vi "HFRR ADV v030 new software.vi"() -> ()   [LabVIEW 2025] (continued)
        n1482 = property on="About" class="Bool (strict)"("DisabledEnum"=w1363) -> ()  [unwired: 2 in, 2 out]
      }
      frame "Test Setup" {
        w1369 = T19."Enabled" ("Disabled")
        n1483 = local read "Service Password enable"() -> (w1368:bool)
        n1484 = property on="Dashboard" class="Bool (strict)"("DisabledEnum"=T19."Disabled" ("Disabled")) -> ()  [unwired: 2 in, 2 out]
        n1485 = property on="Imaging" class="Bool (strict)"("DisabledEnum"=w1369) -> ()  [unwired: 2 in, 2 out]
        n1486 = property on="Analysis" class="Bool (strict)"("DisabledEnum"=w1369) -> ()  [unwired: 2 in, 2 out]
        n1487 = property on="Home" class="Bool (strict)"("DisabledEnum"=w1369) -> ()  [unwired: 2 in, 2 out]
        n1488 = property on="Report" class="Bool (strict)"("DisabledEnum"=w1369) -> ()  [unwired: 2 in, 2 out]
        n1489 = property on="Test Setup" class="Bool (strict)"("DisabledEnum"=w1369) -> ()  [unwired: 2 in, 2 out]
        n1490 = case shown="True" w1368 {
          tunnel: [T19."Disabled" ("Disabled") T19."Enabled" ("Disabled")] -> w1367
          frame False {
          }
          frame True {
          }
        }
        n1491 = property on="About" class="Bool (strict)"("DisabledEnum"=w1367) -> ()  [unwired: 2 in, 2 out]
      }
      frame "Adv Scar" {
        w1376 = T19."Enabled" ("Disabled")
        n1492 = property on="Dashboard" class="Bool (strict)"("DisabledEnum"=T19."Disabled" ("Disabled")) -> ()  [unwired: 2 in, 2 out]
        n1493 = property on="Imaging" class="Bool (strict)"("DisabledEnum"=w1376) -> ()  [unwired: 2 in, 2 out]
        n1494 = property on="Analysis" class="Bool (strict)"("DisabledEnum"=w1376) -> ()  [unwired: 2 in, 2 out]
        n1495 = property on="Home" class="Bool (strict)"("DisabledEnum"=w1376) -> ()  [unwired: 2 in, 2 out]
        n1496 = property on="Report" class="Bool (strict)"("DisabledEnum"=w1376) -> ()  [unwired: 2 in, 2 out]
        n1497 = property on="Test Setup" class="Bool (strict)"("DisabledEnum"=w1376) -> ()  [unwired: 2 in, 2 out]
        n1498 = local read "Service Password enable"() -> (w1374:bool)
        n1499 = case shown="True" w1374 {
          tunnel: [T19."Disabled" ("Disabled") T19."Enabled" ("Disabled")] -> w1373
          frame False {
          }
          frame True {
          }
        }
        n1500 = property on="About" class="Bool (strict)"("DisabledEnum"=w1373) -> ()  [unwired: 2 in, 2 out]
      }
      frame "Calibration" {
        w1379 = T19."Enabled" ("Disabled")
        n1501 = property on="Dashboard" class="Bool (strict)"("DisabledEnum"=T19."Disabled" ("Disabled")) -> ()  [unwired: 2 in, 2 out]
        n1502 = property on="Imaging" class="Bool (strict)"("DisabledEnum"=w1379) -> ()  [unwired: 2 in, 2 out]
        n1503 = property on="Analysis" class="Bool (strict)"("DisabledEnum"=w1379) -> ()  [unwired: 2 in, 2 out]
        n1504 = property on="Home" class="Bool (strict)"("DisabledEnum"=w1379) -> ()  [unwired: 2 in, 2 out]
        n1505 = property on="Report" class="Bool (strict)"("DisabledEnum"=w1379) -> ()  [unwired: 2 in, 2 out]
        n1506 = property on="Test Setup" class="Bool (strict)"("DisabledEnum"=w1379) -> ()  [unwired: 2 in, 2 out]
        n1507 = local read "Service Password enable"() -> (w1381:bool)
        n1508 = property on="Calibration" class="Bool (strict)"("DisabledEnum"=w1379) -> ()  [unwired: 2 in, 2 out]
        n1509 = case shown="True" w1381 {
          tunnel: [T19."Disabled" ("Disabled") T19."Enabled" ("Disabled")] -> w1380
          frame False {
          }
          frame True {
          }
        }
        n1510 = property on="About" class="Bool (strict)"("DisabledEnum"=w1380) -> ()  [unwired: 2 in, 2 out]
      }
      frame "Adv Scar Report" {
        w1387 = T19."Enabled" ("Disabled")
        n1511 = property on="Dashboard" class="Bool (strict)"("DisabledEnum"=T19."Disabled" ("Disabled")) -> ()  [unwired: 2 in, 2 out]
        n1512 = property on="Imaging" class="Bool (strict)"("DisabledEnum"=w1387) -> ()  [unwired: 2 in, 2 out]
        n1513 = property on="Analysis" class="Bool (strict)"("DisabledEnum"=w1387) -> ()  [unwired: 2 in, 2 out]
        n1514 = property on="Home" class="Bool (strict)"("DisabledEnum"=w1387) -> ()  [unwired: 2 in, 2 out]
        n1515 = property on="Report" class="Bool (strict)"("DisabledEnum"=w1387) -> ()  [unwired: 2 in, 2 out]
        n1516 = property on="Test Setup" class="Bool (strict)"("DisabledEnum"=w1387) -> ()  [unwired: 2 in, 2 out]
        n1517 = local read "Service Password enable"() -> (w1386:bool)
        n1518 = case shown="True" w1386 {
          tunnel: [T19."Disabled" ("Disabled") T19."Enabled" ("Disabled")] -> w1385
          frame False {
          }
          frame True {
          }
        }
        n1519 = property on="About" class="Bool (strict)"("DisabledEnum"=w1385) -> ()  [unwired: 2 in, 2 out]
      }
      frame "Compare Files" {
        w1393 = T19."Enabled" ("Disabled")
        n1520 = local read "Service Password enable"() -> (w1392:bool)
        n1521 = property on="Dashboard" class="Bool (strict)"("DisabledEnum"=T19."Disabled" ("Disabled")) -> ()  [unwired: 2 in, 2 out]
        n1522 = property on="Imaging" class="Bool (strict)"("DisabledEnum"=w1393) -> ()  [unwired: 2 in, 2 out]
        n1523 = property on="Analysis" class="Bool (strict)"("DisabledEnum"=w1393) -> ()  [unwired: 2 in, 2 out]
        n1524 = property on="Home" class="Bool (strict)"("DisabledEnum"=w1393) -> ()  [unwired: 2 in, 2 out]
        n1525 = property on="Report" class="Bool (strict)"("DisabledEnum"=w1393) -> ()  [unwired: 2 in, 2 out]
        n1526 = property on="Test Setup" class="Bool (strict)"("DisabledEnum"=w1393) -> ()  [unwired: 2 in, 2 out]
        n1527 = case shown="True" w1392 {
          tunnel: [T19."Disabled" ("Disabled") T19."Enabled" ("Disabled")] -> w1391
          frame False {
          }
          frame True {
          }
        }
        n1528 = property on="About" class="Bool (strict)"("DisabledEnum"=w1391) -> ()  [unwired: 2 in, 2 out]
      }
      frame "Acquire" {
        n1529 = local read "Service Password enable"() -> (w1398:bool)
        n1530 = property on="Test Setup" class="Bool (strict)"("DisabledEnum"=T19."Disabled" ("Disabled")) -> ()  [unwired: 2 in, 2 out]
        n1531 = local read "Auto Start Test"() -> (w1400:bool)
        n1532 = local read "RUN"() -> (w1402:bool)
        n1533 = case shown="True" w1398 {
          tunnel: [T19."Disabled" ("Disabled") T19."Enabled" ("Disabled")] -> w1399
          frame False {
          }
          frame True {
          }
        }
        n1534 = Or(x=w1402, y=w1400) -> (x .or. y?=w1401:bool)
        n1535 = case shown="True" w1401 {
          tunnel: [T19."Enabled" ("Disabled") T19."Disabled" ("Disabled")] -> w1397
          frame False {
          }
          frame True {
          }
        }
        n1536 = property on="About" class="Bool (strict)"("DisabledEnum"=w1399) -> ()  [unwired: 2 in, 2 out]
        n1537 = property on="Imaging" class="Bool (strict)"("DisabledEnum"=w1397) -> ()  [unwired: 2 in, 2 out]
        n1538 = property on="Dashboard" class="Bool (strict)"("DisabledEnum"=w1397) -> ()  [unwired: 2 in, 2 out]
        n1539 = property on="Analysis" class="Bool (strict)"("DisabledEnum"=w1397) -> ()  [unwired: 2 in, 2 out]
        n1540 = property on="Home" class="Bool (strict)"("DisabledEnum"=w1397) -> ()  [unwired: 2 in, 2 out]
        n1541 = property on="Report" class="Bool (strict)"("DisabledEnum"=w1397) -> ()  [unwired: 2 in, 2 out]
        n1542 = property on="Calibration" class="Bool (strict)"("DisabledEnum"=w1397) -> ()  [unwired: 2 in, 2 out]
      }
      frame "About" {
        n1543 = local read "FILE"() -> (w1416:string)
        n1544 = local read "TEST FILE NAM,E SAVED"() -> (w1409:bool)
        n1545 = call <vilib>:"Trim Whitespace.vi"("string"=w1416) -> ("trimmed string"=w1415:string)  [unwired: 1 in]
        n1546 = local read "Auto Start Test"() -> (w1419:bool)
        n1547 = String Length(string=w1415) -> (length=w1414:i32)
        n1548 = Greater?(x=w1414, y=1) -> (0:w1411:bool)
        n1549 = And(x=w1411, y=w1409) -> (x .and. y?=w1410:bool)
        n1550 = local read "RUN"() -> (w1421:bool)
        n1551 = case shown="True" w1410 {
          tunnel: [T19."Disabled" ("Disabled") T19."Enabled" ("Disabled")] -> w1412
          frame False {
          }
          frame True {
          }
        }
        n1552 = Or(x=w1421, y=w1419) -> (x .or. y?=w1420:bool)
        n1553 = property on="About" class="Bool (strict)"("DisabledEnum"=T19."Enabled" ("Disabled")) -> ()  [unwired: 2 in, 2 out]
        n1554 = case shown="False" w1420 {
          tunnel: [T19."Enabled" ("Disabled") T19."Disabled" ("Disabled")] -> w1418
          frame False {
          }
          frame True {
          }
        }
        n1555 = property on="Dashboard" class="Bool (strict)"("DisabledEnum"=w1412) -> ()  [unwired: 2 in, 2 out]
        n1556 = property on="Test Setup" class="Bool (strict)"("DisabledEnum"=T19."Disabled" ("Disabled")) -> ()  [unwired: 2 in, 2 out]
        n1557 = property on="Imaging" class="Bool (strict)"("DisabledEnum"=w1418) -> ()  [unwired: 2 in, 2 out]
        n1558 = property on="Analysis" class="Bool (strict)"("DisabledEnum"=w1418) -> ()  [unwired: 2 in, 2 out]
        n1559 = property on="Home" class="Bool (strict)"("DisabledEnum"=w1418) -> ()  [unwired: 2 in, 2 out]
        n1560 = property on="Report" class="Bool (strict)"("DisabledEnum"=w1418) -> ()  [unwired: 2 in, 2 out]
      }
    }
    n1561 = local read "Quit"() -> (w1346:bool)
    "Single" <- "Single - Graph"
  }
  n1562 = disable-structure shown="Disabled" {
    disable-tunnel: [w1698 _] -> w42
    disable-tunnel: _ -> [w1697 _]
    frame Disabled {
      n1563 = while {
        tunnel: w1697 -> [_]
        tunnel: [w1699] -> w1698
        tunnel: [w1700] -> _
        i -> [w1700]
        stop <- w1699 stop-if-true
        w1716 = u16 10 items=["1.0"=10, "1.5"=15, "2.0"=20] ("stop bits (10: 1 bit)")
        n1564 = Wait (ms)(milliseconds to wait=u32 10) -> ()  [unwired: 1 out]
        n1565 = call-poly "VISA Configure Serial Port"("VISA resource name"=refnum<visa-resource-name> "ASRL1::INSTR" ("COM PORT"), "timeout (10sec)"=u32 10, "baud rate (9600)"=u32 57600, "data bits (8)"=u16 8, "stop bits (10: 1 bit)"=w1716) -> ("VISA resource name out"=w1702:refnum<visa-resource-name>, "error out"=w1711:errorcluster)  [unwired: 9 in]
        n1566 = VISA Read(VISA resource name=w1702, byte count=u32 2 ("byte count (0)")) -> (read buffer=w1710:string)  [unwired: 1 in, 3 out]
        n1567 = String Subset(string=w1710, offset (0)=0, length (rest)=2 ("length (rest)")) -> (substring=w1709:string)
        n1568 = Match Pattern(string=w1709, regular expression="<>") -> (offset past match=w1706:i32)  [unwired: 1 in, 3 out]
        n1569 = Greater Or Equal?(x=w1706, y=0) -> (x >= y?=w1701:bool)
        n1570 = case shown="True" w1701 {
          tunnel: w1702 -> [_ w1720]
          tunnel: w1711 -> [_ w1719]
          frame False {
          }
          frame True {
            n1571 = VISA Read(VISA resource name=w1720, byte count=u32 32 ("byte count (0)"), error in (no error)=w1719) -> (read buffer=w1718:string)  [unwired: 3 out]
            n1572 = String Subset(string=w1718, offset (0)=0, length (rest)=8 ("length (rest)")) -> (substring=w1722:string)
            n1573 = String Subset(string=w1718, offset (0)=8, length (rest)=8 ("length (rest)")) -> (substring=w1723:string)
            n1574 = Decimal String To Number(string=w1723) -> (number=w1730:i32)  [unwired: 2 in, 1 out]
            n1575 = Decimal String To Number(string=w1722) -> (number=w1726:i32)  [unwired: 2 in, 1 out]
            n1576 = Divide(x=w1730, y=10000) -> ()  [unwired: 1 out]
            n1577 = Divide(x=w1726, y=1000000) -> ()  [unwired: 1 out]
          }
        }
        n1578 = local read "Quit"() -> (w1699:bool)
      }
    }
    frame Enabled {
    }
  }
  n1579 = Tick Count (ms)() -> (millisecond timer value=w4:u32)
  n1580 = while {
    shift-right: [w1776] -> _
    shift-left: w6 -> [w1780]
    shift-right: [w1775] -> _
    shift-left: w5 -> [w1779]
    shift-right: [w1774] -> _
    shift-left: w6 -> [w1778]
    shift-right: [w1773] -> _
    shift-left: w5 -> [w1777]
    shift-right: [w1771] -> _
    shift-left: w4 -> [w1772]
    shift-right: [w1768] -> _
    shift-left: w3 -> [w1769]
    shift-right: [w1767] -> _
    shift-left: w3 -> [w1770]
    shift-right: [w1760] -> _
    shift-left: w3 -> [w1766]
    shift-right: [w1759] -> _
    shift-left: w3 -> [w1765]
    shift-right: [w1758] -> _
    shift-left: w3 -> [w1764]
    shift-right: [w1757] -> _
    shift-left: w3 -> [w1763]
    shift-right: [w1756] -> _
    shift-left: w3 -> [w1762]
    shift-right: [w1755] -> _
    shift-left: w3 -> [w1761]
    shift-right: [w1754] -> _
    shift-left: w3 -> [w1748]
    shift-right: [w1753] -> _
    shift-left: w3 -> [w1747]
    shift-right: [w1752] -> _
    shift-left: w3 -> [w1746]
    shift-right: [w1751] -> _
    shift-left: w3 -> [w1745]
    shift-right: [w1750] -> _
    shift-left: w3 -> [w1744]
    shift-right: [w1749] -> _
    shift-left: w3 -> [w1743]
    shift-right: [w1734] -> _
    shift-left: w3 -> [w1737]
    shift-right: [w1733] -> _
    shift-left: w3 -> [w1736]
    shift-right: [w1732] -> _
    shift-left: w3 -> [w1735]
    stop <- w1782 stop-if-true
    n1581 = local read "Read UNO"() -> (w1741:string)
    n1582 = local read "Error  2"() -> (w1781:errorcluster)
    n1583 = String Length(string=w1741) -> (length=w1740:i32)
    n1584 = call <vilib>:"Trim Whitespace.vi"("string"=w1741) -> ("trimmed string"=w1742:string)  [unwired: 1 in]
    n1585 = Greater Or Equal?(x=w1740, y=23) -> (x >= y?=w1738:bool)
    n1586 = case shown="No Error" w1781 {
      tunnel: w1780 -> [w1828 w1924]
      tunnel: w1779 -> [w1827 w1923]
      tunnel: w1778 -> [w1826 w1922]
      tunnel: w1777 -> [w1825 w1921]
      tunnel: [w1824 w1924] -> w1776
      tunnel: [w1823 w1923] -> w1775
      tunnel: [w1822 w1922] -> w1774
      tunnel: [w1821 w1921] -> w1773
      tunnel: w1772 -> [w1820 w1920]
      tunnel: [w1819 w1920] -> w1771
      tunnel: w1769 -> [w1818 w1919]
      tunnel: w1770 -> [w1817 w1918]
      tunnel: [w1816 w1919] -> w1768
      tunnel: [w1815 w1918] -> w1767
      tunnel: w1766 -> [w1814 w1917]
      tunnel: w1765 -> [w1813 w1916]
      tunnel: w1764 -> [w1812 w1915]
      tunnel: w1763 -> [w1811 w1914]
      tunnel: w1762 -> [w1810 w1913]
      tunnel: w1761 -> [w1809 w1912]
      tunnel: [w1808 w1917] -> w1760
      tunnel: [w1807 w1916] -> w1759
      tunnel: [w1806 w1915] -> w1758
      tunnel: [w1805 w1914] -> w1757
      tunnel: [w1804 w1913] -> w1756
      tunnel: [w1803 w1912] -> w1755
      tunnel: w1748 -> [w1802 w1911]
      tunnel: [w1801 w1911] -> w1754
      tunnel: [w1800 w1907] -> w1753
      tunnel: [w1799 w1906] -> w1752
      tunnel: [w1798 w1910] -> w1751
      tunnel: [w1797 w1909] -> w1750
      tunnel: [w1796 w1908] -> w1749
      tunnel: w1747 -> [w1795 w1910]
      tunnel: w1746 -> [w1794 w1909]
      tunnel: w1745 -> [w1793 w1908]
      tunnel: w1744 -> [w1792 w1907]
      tunnel: w1743 -> [w1791 w1906]
      tunnel: w1742 -> [w1790 _]
      tunnel: w1738 -> [w1789 _]
      tunnel: w1737 -> [w1788 w1905]
      tunnel: w1736 -> [w1787 w1904]
      tunnel: w1735 -> [w1786 w1903]
      tunnel: [w1785 w1905] -> w1734
      tunnel: [w1784 w1904] -> w1733
      tunnel: [w1783 w1903] -> w1732
      frame No Error {
        n1587 = case shown="True" w1789 {
          tunnel: w1828 -> [w1844 w1896]
          tunnel: w1827 -> [w1843 w1895]
          tunnel: w1826 -> [w1842 w1894]
          tunnel: w1825 -> [w1841 w1893]
          tunnel: [w1844 w1892] -> w1824
          tunnel: [w1843 w1891] -> w1823
          tunnel: [w1842 w1890] -> w1822
          tunnel: [w1841 w1889] -> w1821
          tunnel: w1820 -> [w1840 w1887]
          tunnel: [w1840 w1886] -> w1819
          tunnel: w1818 -> [w1839 w1885]
          tunnel: w1817 -> [w1838 w1884]
          tunnel: [w1839 w1883] -> w1816
          tunnel: [w1838 w1882] -> w1815
          tunnel: w1814 -> [w1837 w1881]
          tunnel: w1813 -> [w1836 w1880]
          tunnel: w1812 -> [w1835 w1879]
          tunnel: w1811 -> [w1834 w1878]
          tunnel: w1810 -> [w1833 w1877]
          tunnel: w1809 -> [w1832 w1876]
          tunnel: [w1837 w1875] -> w1808
          tunnel: [w1836 w1874] -> w1807
          tunnel: [w1835 w1873] -> w1806
          tunnel: [w1834 w1872] -> w1805
          tunnel: [w1833 w1871] -> w1804
          tunnel: [w1832 w1870] -> w1803
          tunnel: w1802 -> [w1850 w1869]
          tunnel: [w1850 w1868] -> w1801
          tunnel: [w1847 w1867] -> w1800
          tunnel: [w1846 w1866] -> w1799
          tunnel: [w1849 w1865] -> w1798
          tunnel: [w1845 w1864] -> w1797
          tunnel: [w1848 w1863] -> w1796
          tunnel: w1795 -> [w1849 w1862]
          tunnel: w1794 -> [w1848 w1861]
          tunnel: w1793 -> [w1847 w1860]
          tunnel: w1792 -> [w1846 w1859]
          tunnel: w1791 -> [w1845 w1858]
          tunnel: w1790 -> [_ w1857]
          tunnel: w1788 -> [w1831 w1856]
          tunnel: w1787 -> [w1830 w1855]
          tunnel: w1786 -> [w1829 w1854]
          tunnel: [w1831 w1853] -> w1785
          tunnel: [w1830 w1852] -> w1784
          tunnel: [w1829 w1851] -> w1783
          frame False {
          }
          frame True {
            n1588 = Tick Count (ms)() -> (millisecond timer value=w1888:u32)
            n1589 = String To Byte Array(string=w1857) -> (unsigned byte array=w1901:u8[])
            n1590 = Array Size(array=w1901) -> (size(s)=w1900:i32)
            n1591 = formula code="// --- INTERNAL VARIABLE DECLARATIONS ---\nint i = 0;\nint k = 0;\nint start_idx = -1;\nint end_idx = -1;\nint phase = 0;\nint sign0 = 1;\nint sign1 = 1;\nint ch0_val = 0;   \nint ch1_val = 0;   \nfloat ch0_raw = 0.0;\nfloat ch1_raw = 0.0;\nfloat temp0 = 0.0;\nfloat temp1 = 0.0;\nfloat ch0_clean = 0.0;\nfloat ch1_clean = 0.0;\n\n// Temporal intermediate variables for calculation smoothing\nfloat raw_p2p_v = 0.0;\nfloat raw_friction = 0.0;\nfloat raw_cof = 0.0;\n\n// Temporal intermediate variables for Piezo voltage translations\nfloat piezo_min_v = 0.0;\nfloat piezo_max_v = 0.0;\n\n// Initialize output variables to current shift register states right away\nout_LVDT_Min_V = in_LVDT_Min_V;\nout_LVDT_Max_V = in_LVDT_Max_V;\nout_LVDT_P2P_V = in_LVDT_P2P_V;\nout_Piezo_P2P = in_Piezo_P2P;\nout_Friction_N = in_Friction_N;\nout_COF = in_COF;\nwindow_ready = 0;\n\n// --- STEP 1: PARSE EVERY STRING IN THE BYTE ARRAY ---\nif (array_size > 2) {\n    for (i = 0; i < array_size - 1; i++) {\n        if (raw_bytes[i] == 42) { // '*' character detected\n            start_idx = i;\n        }\n        \n        // Match standard delimiter sequence \";&\" or end window character\n        if (raw_bytes[i] == 59 && raw_bytes[i+1] == 38 && start_idx != -1) { \n            end_idx = i;\n            ch0_val = 0;\n            ch1_val = 0;\n            sign0 = 1;\n            sign1 = 1;\n            phase = 0; \n\n            for (k = start_idx + 1; k < end_idx; k++) {\n                if (raw_bytes[k] == 45) { // '-' sign\n                    if (phase == 0) sign0 = -1;\n                    else sign1 = -1;\n                }\n                else if (raw_bytes[k] == 43) { // '+' sign\n                    if (phase == 0) sign0 = 1;\n                    else sign1 = 1;\n                }\n                else if (raw_bytes[k] == 59) { // ';' delimiter\n                    phase = 1; \n                }\n                else if (raw_bytes[k] >= 48 && raw_bytes[k] <= 57) { // Numeric ASCII digits\n                    if (phase == 0) {\n                        ch0_val = (ch0_val * 10) + (raw_bytes[k] - 48);\n                    } else {\n                        ch1_val = (ch1_val * 10) + (raw_bytes[k] - 48);\n                    }\n                }\n            }\n\n            // Implicit type conversion\n            ch0_raw = ch0_val * sign0 * 1.0;\n            ch1_raw = ch1_val * sign1 * 1.0;\n\n            // --- STEP 2: 3-SAMPLE MEDIAN FILTER ---\n            m0_2 = m0_1; m0_1 = m0_0; m0_0 = ch0_raw;\n            float s0_0 = m0_0; float s0_1 = m0_1; float s0_2 = m0_2;\n            if (s0_0 > s0_1) { temp0 = s0_0; s0_0 = s0_1; s0_1 = temp0; }\n            if (s0_1 > s0_2) { temp0 = s0_1; s0_1 = s0_2; s0_2 = temp0; }\n            if (s0_0 > s0_1) { temp0 = s0_0; s0_0 = s0_1; s0_1 = temp0; }\n            ch0_clean = s0_1;\n\n            m1_2 = m1_1; m1_1 = m1_0; m1_0 = ch1_raw;\n            float s1_0 = m1_0; float s1_1 = m1_1; float s1_2 = m1_2;\n            if (s1_0 > s1_1) { temp1 = s1_0; s1_0 = s1_1; s1_1 = temp1; }\n            if (s1_1 > s1_2) { temp1 = s1_1; s1_1 = s1_2; s1_2 = temp1; }\n            if (s1_0 > s1_1) { temp1 = s1_0; s1_0 = s1_1; s1_1 = temp1; }\n            ch1_clean = s1_1;\n\n            // --- STEP 3: EXPONENTIAL FILTER (STREAM LEVEL) ---\n            if (ch0_filt == 0.0) ch0_filt = ch0_clean;\n            if (ch1_filt == 0.0) ch1_filt = ch1_clean;\n\n            ch0_filt = ch0_filt + (ch0_clean - ch0_filt) * 0.125;\n            ch1_filt = ch1_filt + (ch1_clean - ch1_filt) * 0.125;\n\n            // --- STEP 4: MIN/MAX WINDOW CONTINUOUS ACCUMULATION ---\n            if (ch0_filt > max_ch0) max_ch0 = ch0_filt;\n            if (ch0_filt < min_ch0) min_ch0 = ch0_filt;\n            if (ch1_filt > max_ch1) max_ch1 = ch1_filt;\n            if (ch1_filt < min_ch1) min_ch1 = ch1_filt;\n\n            start_idx = -1; \n        }\n    }\n}\n\n// --- STEP 5: WINDOW EVALUATION ENGINE ---\nif (((current_time_ms - start_time_ms) >= 50) && (min_ch0 < 9000000.0) && (max_ch0 > -9000000.0)) {\n    window_ready = 1;\n\n    // Linear Bit-to-Voltage Transformations (LVDT - Channel 0)\n    out_LVDT_Min_V = (min_ch0 * VREF) / 8388607.0;\n    out_LVDT_Max_V = (max_ch0 * VREF) / 8388607.0;\n    raw_p2p_v = out_LVDT_Max_V - out_LVDT_Min_V;\n\n    // Linear Bit-to-Voltage Transformations (Piezo - Channel 1)\n    piezo_min_v = (min_ch1 * VREF) / 8388607.0;\n    piezo_max_v = (max_ch1 * VREF) / 8388607.0;\n    \n    // Assign Peak-to-Peak Voltage directly to output indicator (Matches Python logic)\n    out_Piezo_P2P = piezo_max_v - piezo_min_v;\n    \n    // Force scaling calculations using Voltage delta * Newtons/Volt Factor\n    raw_friction = out_Piezo_P2P * PIEZO_CAL_FACTOR+0.44528;\n    raw_cof = raw_friction / NORMAL_FORCE;\n\n    // --- STEP 6: OUTPUT METRIC SMOOTHING (Low-Pass Filter Alpha = 0.05) ---\n    // Seed initial historical metrics if first loop iteration\n    if (hist_LVDT_P2P == 0.0) hist_LVDT_P2P = raw_p2p_v;\n    if (hist_Friction == 0.0) hist_Friction = raw_friction;\n    if (hist_COF == 0.0)      hist_COF = raw_cof;\n\n    // Apply exponential output dampening\n    hist_LVDT_P2P = hist_LVDT_P2P + (raw_p2p_v - hist_LVDT_P2P) * 0.05;\n    hist_Friction = hist_Friction + (raw_friction - hist_Friction) * 0.05;\n    hist_COF      = hist_COF + (raw_cof - hist_COF) * 0.05;\n\n    // Direct smoothed parameters out to UI Indicators\n    out_LVDT_P2P_V = hist_LVDT_P2P;\n    out_Friction_N = hist_Friction;\n    out_COF        = hist_COF;\n\n    // Reset tracking targets to extreme boundaries safely\n    min_ch0 = 9999999.0;\n    max_ch0 = -9999999.0;\n    min_ch1 = 9999999.0;\n    max_ch1 = -9999999.0;\n\n    start_time_ms = current_time_ms;\n}"("raw_bytes"=w1901, "array_size"=w1900, "VREF"="VREF", "PIEZO_CAL_FACTOR"="PIEZO_CAL_FACTOR", "NORMAL_FORCE"="NORMAL_FORCE", "min_ch0"=w1896, "max_ch0"=w1895, "min_ch1"=w1894, "max_ch1"=w1893, "current_time_ms"=w1888, "start_time_ms"=w1887, "ch0_filt"=w1885, "ch1_filt"=w1884, "m0_0"=w1881, "m0_1"=w1880, "m0_2"=w1879, "m1_0"=w1878, "m1_1"=w1877, "m1_2"=w1876, "in_LVDT_Min_V"=w1869, "in_LVDT_Max_V"=w1862, "in_LVDT_P2P_V"=w1861, "in_Piezo_P2P"=w1860, "in_Friction_N"=w1859, "in_COF"=w1858, "hist_LVDT_P2P"=w1856, "hist_Friction"=w1855, "hist_COF"=w1854) -> ("window_ready"=→"Valid_data":dbl, "out_LVDT_Min_V"=w1868:dbl, "out_LVDT_Max_V"=w1867:dbl, "out_LVDT_P2P_V"=w1866:dbl, "out_Piezo_P2P"=w1865:dbl, "out_Friction_N"=w1864:dbl, "out_COF"=w1863:dbl, "min_ch0"=w1892:dbl, "max_ch0"=w1891:dbl, "min_ch1"=w1890:dbl, "max_ch1"=w1889:dbl, "start_time_ms"=w1886:u32, "ch0_filt"=w1883:dbl, "ch1_filt"=w1882:dbl, "m0_0"=w1875:dbl, "m0_1"=w1874:dbl, "m0_2"=w1873:dbl, "m1_0"=w1872:dbl, "m1_1"=w1871:dbl, "m1_2"=w1870:dbl, "hist_LVDT_P2P"=w1853:dbl, "hist_Friction"=w1852:dbl, "hist_COF"=w1851:dbl)
            "LVDT MIN" <- w1868
            "LVDT MAX" <- w1867
            "LVDT Peak" <- w1866
            "pizo raw" <- w1865
            "Friction" <- w1864
            "cof" <- w1863
          }
        }
      }
      frame Error {
      }
    }
    n1592 = local read "Quit"() -> (w1782:bool)
  }
  n1593 = disable-structure shown="Disabled" {
    disable-tunnel: errorcluster {"status"=TRUE, "code"=0, "source"="Init"} ("error IO") -> [w1927 _]
    disable-tunnel: [w1925 _] -> w45
    frame Disabled {
      n1594 = while {
        shift-right: [w1943] -> w1929
        shift-left: _ -> [w1934]
        shift-right: [w1942] -> w1928
        shift-left: w1927 -> [w1936]
        tunnel: [w1931] -> w1925
        tunnel: [w1941] -> _
        i -> [w1941]
        stop <- w1931 stop-if-true
        n1595 = local read "Port 1a"() -> (w1937:bool)
        n1596 = local read "Port 3"() -> (w1938:bool)
        n1597 = local read "Com Port 1"() -> (w1935:refnum<visa-resource-name>)
        n1598 = Or(x=w1938, y=w1937) -> (x .or. y?=w1940:bool)
        n1599 = Unbundle(w1936) -> ("status"=→"Port 3":bool)  [unwired: 2 out]
        n1600 = Not Equal?(x=w1935, y=w1934) -> (x != y?=w1932:bool)
        n1601 = case shown="True" w1940 {
          frame False {
            w1946 = TRUE ("Visible")
            n1602 = property on="Port 1a" class="Bool (strict)"("Visible"=w1946) -> ()  [unwired: 2 in, 2 out]
            n1603 = property on="Port 3" class="Bool (strict)"("Visible"=w1946) -> ()  [unwired: 2 in, 2 out]
          }
          frame True {
            w1947 = TRUE ("Visible")
            n1604 = property on="Port 1a" class="Bool (strict)"("Visible"=w1947) -> ()  [unwired: 2 in, 2 out]
            n1605 = property on="Port 3" class="Bool (strict)"("Visible"=w1947) -> ()  [unwired: 2 in, 2 out]
          }
        }
        n1606 = Wait (ms)(milliseconds to wait=u32 40) -> ()  [unwired: 1 out]
        n1607 = case shown="True" w1932 {
          tunnel: [w1944 errorcluster {"status"=TRUE, "code"=0, "source"="Init"} ("error out")] -> w1933
          tunnel: w1936 -> [w1944 _]
          frame False {
          }
          frame True {
          }
        }
        n1608 = case shown="Error" w1933 {
          selector: w1933 -> [w1954 w1972]
          tunnel: [w1957 w1976] -> w1943
          tunnel: [w1956 w1970] -> w1942
          tunnel: w1934 -> [w1955 w1974]
          frame No Error {
            n1609 = property class="Instr"(reference=w1955, error in=w1954) -> (reference out=w1952:refnum<visa-resource-name>, error out=w1953:errorcluster, "Serial Settings:Number of Bytes at Serial Port"=w1949:u32)
            n1610 = Greater?(x=w1949, y=u32 5) -> (0:w1948:bool)
            n1611 = Not(x=w1948) -> (.not. x?=→"Port 1a":bool)
            n1612 = while {
              tunnel: [w1965] -> w1956
              tunnel: [w1964] -> w1957
              tunnel: w1953 -> [w1963]
              tunnel: w1952 -> [w1962]
              stop <- TRUE stop-if-true
              n1613 = property class="Instr" props=["Serial Settings:Number of Bytes at Serial Port"](reference=w1962, error in=w1963) -> (reference out=w1967:refnum<visa-resource-name>, error out=w1966:errorcluster)  [unwired: 1 out]
              n1614 = VISA Read(VISA resource name=w1967, byte count=u32 50, error in (no error)=w1966) -> (VISA resource name out=w1964:refnum<visa-resource-name>, read buffer=w1959:string, error out=w1965:errorcluster)  [unwired: 1 out]
              n1615 = Wait (ms)(milliseconds to wait=u32 5) -> ()  [unwired: 1 out]
            }
          }
          frame Error {
            w1982 = u16 0 items=["None", "XON/XOFF", "RTS/CTS", "XON/XOFF & RTS/CTS", "DTR/DSR", "XON/XOFF & DTR/DSR"] ("flow control (0:none)  2")
            w1980 = u16 10 items=["1.0"=10, "1.5"=15, "2.0"=20] ("stop bits 2")
            w1978 = u16 0 items=["None", "Odd", "Even", "Mark", "Space"] ("parity 2")
            w1979 = u32 10000  # timeout (10sec)
            n1616 = VISA Close(VISA resource name=w1974, error in (no error)=w1972) -> (error out=w1975:errorcluster)
            n1617 = local write "Port 1a"(FALSE ("Port 1a")) -> ()
            n1618 = local read "Com Port 1"() -> (w1969:refnum<visa-resource-name>)
            n1619 = call <vilib>:"Clear Errors.vi"("error in (no error)"=w1975) -> ("error out"=w1973:errorcluster)  [unwired: 5 in, 1 out]
            n1620 = call-poly "VISA Configure Serial Port"("VISA resource name"=w1969, "timeout (10sec)"=w1979, "baud rate (9600)"=u32 250000 ("baud rate  2"), "data bits (8)"=u16 8 ("data bits  2"), "parity (0:none)"=w1978, "error in (no error)"=w1973, "stop bits (10: 1 bit)"=w1980, "flow control (0:none)"=w1982) -> ("VISA resource name out"=w1983:refnum<visa-resource-name>, "error out"=w1984:errorcluster)  [unwired: 6 in]
            n1621 = flat-sequence {
              tunnel: w1983 -> [w1986]
              tunnel: w1984 -> [w1985]
              tunnel: [w1986] -> w1976
              tunnel: [w1985] -> w1970
              frame #0 {
                n1622 = Wait (ms)(milliseconds to wait=u32 50) -> ()  [unwired: 1 out]
              }
            }
            "Residual Uno" <- ""
          }
        }
        n1623 = local read "Quit"() -> (w1931:bool)
        "Error Uno" <- w1936
      }
      n1624 = VISA Close(VISA resource name=w1929, error in (no error)=w1928) -> (error out=w1926:errorcluster)
      n1625 = call <vilib>:"Clear Errors.vi"("error in (no error)"=w1926) -> ()  [unwired: 5 in, 2 out]
    }
    frame Enabled {
    }
  }
  n1626 = while {
    stop <- w1997 stop-if-true
    # "V0OLTAGE TO STROKE (peice vise calibration)"
    n1627 = local read "LVDT MIN"() -> (w1989:dbl)
    n1628 = local read "LVDT Peak"() -> (w1988:dbl)
    n1629 = Wait (ms)(milliseconds to wait=u32 10) -> ()  [unwired: 1 out]
    n1630 = formula code="// Dynamic Parameterized Linear Interpolation Node\n// Inputs: vpp_val, voltages (Array), distances (Array)\n// Outputs: stroke\n\nint i = 0;\nint segments = 11; // 12 points make 11 interpolation segments\n\n// 1. Lower Boundary Clamp\nif (vpp_val <= voltages[0]) {\n    stroke = distances[0];\n}\n// 2. Upper Boundary Clamp\nelse if (vpp_val >= voltages[segments]) {\n    stroke = distances[segments];\n}\n// 3. Dynamic Segment Search Loop\nelse {\n    stroke = distances[0]; // Fallback baseline\n    for (i = 0; i < segments; i++) {\n        if (vpp_val >= voltages[i] && vpp_val <= voltages[i+1]) {\n            // Standard linear interpolation formula using array lookups\n            stroke = distances[i] + (vpp_val - voltages[i]) * (distances[i+1] - distances[i]) / (voltages[i+1] - voltages[i]);\n            break; // Segment found, safely exit the loop\n        }\n    }\n}"("vpp_val"=w1988, "voltages"="calibration values", "distances"="STROKE") -> ("stroke"=→"LVDT STROKE":dbl)
    n1631 = local read "Calibration Tare Value"() -> (w1993:dbl)
    n1632 = local read "Calibration Tare"() -> (w1991:bool)
    n1633 = Subtract(x=w1989, y=w1993) -> (x-y=→"LVDT STROKE  Calibration":dbl)
    n1634 = case shown="True" w1991 {
      selector: w1991 -> [_ w1999]
      tunnel: w1989 -> [_ w2000]
      frame False {
      }
      frame True {
        n1635 = Not(x=w1999) -> (.not. x?=w1998:bool)
        n1636 = local write "Calibration Tare"(w1998) -> ()
        "Calibration Tare Value" <- w2000
      }
    }
    n1637 = local read "Quit"() -> (w1997:bool)
  }
  n1638 = while {
    stop <- w2020 stop-if-true
    n1639 = call <vilib>:"High Resolution Polling Wait.vi"("seconds to wait"=0.02) -> ()  [unwired: 10 in, 1 out]
    n1640 = local read "Due read"() -> (w2018:string)
    n1641 = Spreadsheet String To Array(delimiter (Tab)=";", format string="", spreadsheet string=w2018, array type (2D Dbl)=string[] []) -> (array=w2015:string[])
    n1642 = Fract/Exp String To Number(string=w2015) -> (number=w2014:dbl[])  [unwired: 3 in, 1 out]
    n1643 = Index Array(array=w2014) -> (element #1=→"Sample Temperature":dbl, element #2=→"Target Sample Temperature":dbl, element #3=→"Current Duty Cycle":dbl, element #4=→"Ambient Temperature":dbl, element #5=→"Dac Status":dbl, element #6=→"Vpp":dbl, element #7=→"Active Error Code":dbl, element #8=→"Kp":dbl, element #9=→"Ki":dbl, element #10=→"Kd":dbl, element #11=→"SampleRaw":dbl, element #12=→"AmbRaw":dbl)  [unwired: 12 in]
    n1644 = local read "Quit"() -> (w2020:bool)
  }
  n1645 = while {
    shift-right: [w2034] -> w41
    shift-left: _ -> [w2026]
    shift-right: [w2021] -> w40
    shift-left: errorcluster {"status"=FALSE, "code"=0, "source"="Init"} ("error out") -> [w2028]
    tunnel: [w2023] -> w44
    tunnel: [w2033] -> _
    i -> [w2033]
    stop <- w2023 stop-if-true
    n1646 = local read "Com Port 2"() -> (w2027:refnum<visa-resource-name>)
    n1647 = local read "Port 2a"() -> (w2029:bool)
    n1648 = Unbundle(w2028) -> ("status"=→"Port 4":bool)  [unwired: 2 out]
    n1649 = call <vilib>:"High Resolution Polling Wait.vi"("seconds to wait"=0.02) -> ()  [unwired: 10 in, 1 out]
    n1650 = local read "Port 4"() -> (w2030:bool)
    n1651 = Not Equal?(x=w2027, y=w2026) -> (x != y?=w2025:bool)
    n1652 = Or(x=w2030, y=w2029) -> (x .or. y?=w2032:bool)
    n1653 = case shown="False" w2032 {
      frame False {
        w2037 = TRUE ("Visible")
        n1654 = property on="Port 2a" class="Bool (strict)"("Visible"=w2037) -> ()  [unwired: 2 in, 2 out]
        n1655 = property on="Port 4" class="Bool (strict)"("Visible"=w2037) -> ()  [unwired: 2 in, 2 out]
      }
      frame True {
        w2038 = TRUE ("Visible")
        n1656 = property on="Port 2a" class="Bool (strict)"("Visible"=w2038) -> ()  [unwired: 2 in, 2 out]
        n1657 = property on="Port 4" class="Bool (strict)"("Visible"=w2038) -> ()  [unwired: 2 in, 2 out]
      }
    }
    n1658 = case shown="True" w2025 {
      tunnel: [w2035 errorcluster {"status"=TRUE, "code"=0, "source"="Init"} ("error out")] -> w2024
      tunnel: w2028 -> [w2035 _]
      frame False {
      }
      frame True {
      }
    }
    n1659 = case shown="No Error" w2024 {
      selector: w2024 -> [w2051 w2082]
      tunnel: [w2044 w2087] -> w2034
      tunnel: [w2052 w2080] -> w2021
      tunnel: w2026 -> [w2053 w2085]
      frame No Error {
        n1660 = property class="Instr" props=["Serial Settings:Number of Bytes at Serial Port"](reference=w2053, error in=w2051) -> (reference out=w2045:refnum<visa-resource-name>, error out=w2050:errorcluster)  [unwired: 1 out]
        n1661 = while {
          tunnel: [w2061] -> w2046
          tunnel: [w2060] -> w2047
          tunnel: w2050 -> [w2059]
          tunnel: w2045 -> [w2058]
          tunnel: [w2057] -> _
          i -> [w2057]
          stop <- TRUE stop-if-true
          n1662 = property class="Instr" props=["Serial Settings:Number of Bytes at Serial Port"](reference=w2058, error in=w2059) -> (reference out=w2063:refnum<visa-resource-name>, error out=w2062:errorcluster)  [unwired: 1 out]
          n1663 = VISA Read(VISA resource name=w2063, byte count=u32 1000, error in (no error)=w2062) -> (VISA resource name out=w2060:refnum<visa-resource-name>, read buffer=→"Due read":string, error out=w2061:errorcluster)  [unwired: 1 out]
        }
        n1664 = local read "Due Write"() -> (w2043:string)
        n1665 = call <vilib>:"Trim Whitespace.vi"("string"=w2043) -> ("trimmed string"=w2042:string)  [unwired: 1 in]
        n1666 = Not Equal?(x=w2042, y="") -> (x != y?=w2048:bool)
        n1667 = VISA Flush I/O Buffer(VISA resource name=w2047) -> (VISA resource name out=w2040:refnum<visa-resource-name>, error out=→"error out 10":errorcluster)  [unwired: 2 in]
        n1668 = case shown="True" w2048 {
          tunnel: w2040 -> [w2065 w2070]
          tunnel: [w2065 w2074] -> w2044
          tunnel: w2046 -> [w2064 w2069]
          tunnel: [w2064 w2072] -> w2052
          tunnel: w2042 -> [_ w2068]
          tunnel: [_ w2071] -> _
          frame False {
            # "DATA  WRITE LOOP"
          }
          frame True {
            n1669 = Concatenate Strings(w2068, "\r\n") -> (w2067:string)
            n1670 = VISA Write(VISA resource name=w2070, write buffer=w2067, error in (no error)=w2069) -> (VISA resource name out=w2074:refnum<visa-resource-name>, return count=w2071:u32, error out=w2073:errorcluster)
            n1671 = flat-sequence {
              tunnel: w2073 -> [w2076]
              tunnel: [w2076] -> w2072
              frame #0 {
                n1672 = local write "Due Write"("" ("Command")) -> ()
                n1673 = Wait (ms)(milliseconds to wait=u32 5) -> ()  [unwired: 1 out]
              }
            }
          }
        }
        "Port 2a" <- TRUE ("Port 2a")
      }
      frame Error {
        w2093 = u16 0 items=["None", "XON/XOFF", "RTS/CTS", "XON/XOFF & RTS/CTS", "DTR/DSR", "XON/XOFF & DTR/DSR"] ("flow control (0:none)  2")
        w2091 = u16 10 items=["1.0"=10, "1.5"=15, "2.0"=20] ("stop bits 2")
        w2089 = u16 0 items=["None", "Odd", "Even", "Mark", "Space"] ("parity 2")
        w2090 = u32 10000  # timeout (10sec)
        n1674 = VISA Clear(VISA resource name=w2085, error in (no error)=w2082) -> (VISA resource name out=w2084:refnum<visa-resource-name>, error out=w2083:errorcluster)
        n1675 = VISA Close(VISA resource name=w2084, error in (no error)=w2083) -> (error out=w2086:errorcluster)
        n1676 = call <vilib>:"Clear Errors.vi"("error in (no error)"=w2086) -> ()  [unwired: 5 in, 2 out]
        n1677 = local write "Port 2a"(FALSE ("Port 2a")) -> ()
        n1678 = local read "Com Port 2"() -> (w2079:refnum<visa-resource-name>)
        "visa due" <- w2079
        n1679 = call-poly "VISA Configure Serial Port"("VISA resource name"=w2079, "timeout (10sec)"=w2090, "baud rate (9600)"=u32 250000 ("baud rate  2"), "data bits (8)"=u16 8 ("data bits  2"), "parity (0:none)"=w2089, "stop bits (10: 1 bit)"=w2091, "flow control (0:none)"=w2093) -> ("VISA resource name out"=w2094:refnum<visa-resource-name>, "error out"=w2095:errorcluster)  [unwired: 7 in]
        n1680 = flat-sequence {
          tunnel: w2094 -> [w2097]
          tunnel: w2095 -> [w2096]
          tunnel: [w2097] -> w2087
          tunnel: [w2096] -> w2080
          frame #0 {
            n1681 = Wait (ms)(milliseconds to wait=u32 50) -> ()  [unwired: 1 out]
          }
        }
        "Residual Due" <- ""
      }
    }
    "error out 9" <- w2021
    n1682 = local read "Quit"() -> (w2023:bool)
    "Error Due" <- w2028
  }
  n1683 = local write "FRICVALZ"(0.0 ("FRICVALZ")) -> ()
  n1684 = property on="RUN" class="Bool (strict)"("Visible"=TRUE) -> ()  [unwired: 2 in, 2 out]
  n1685 = while {
    tunnel: [w2112] -> _
    tunnel: [w2099] -> w54
    i -> [w2112]
    stop <- w2099 stop-if-true
    n1686 = local read "conststatus"() -> (w2103:dbl)
    n1687 = local read "Main Tab"() -> (w2101:T2)
    n1688 = local read "EDIT"() -> (w2118:bool)
    n1689 = local read "Rate"() -> (w2117:dbl)
    n1690 = case shown="True" w2118 {
      tunnel: [FALSE TRUE] -> _
      frame False {
      }
      frame True {
      }
    }
    n1691 = Equal?(x=w2101, y=T27."About" ("Main Tab")) -> (x = y?=w2110:bool)
    n1692 = Equal?(x=w2103, y=0.0) -> (x = y?=w2104:bool)
    n1693 = Divide(x=1.0, y=w2117) -> (x/y=w2113:dbl)
    "Time 2" <- w2113
    n1694 = case shown="True" w2104 {
      frame False {
      }
      frame True {
        # "C:\\WinDucom\\calibrate WO 2391.dcf"
        n1695 = local write "Lan flag"(22) -> ()
        n1696 = local write "conststatus"(10.0 ("rpm value : 2")) -> ()
        n1697 = String To Path(string="C:\\LAB-IQ\\calibrate WO 2465.dcf") -> (path=w2124:path)
        n1698 = Open/Create/Replace File "Open File"(file path (use dialog)=w2124) -> (refnum out=w2122:refnum<file>)  [unwired: 5 in, 2 out]
        n1699 = for {
          N: 23 -> [_]
          tunnel: w2122 -> [w2133]
          i -> [w2127]
          (unwired) TRUE ("line mode (F)")
          n1700 = Read from Text File "Read File"(file (use dialog)=w2133) -> (text=w2132:string)  [unwired: 3 in, 3 out]
          n1701 = Match Pattern(string=w2132, regular expression="]") -> (after substring=w2130:string)  [unwired: 1 in, 3 out]
          n1702 = String Subset(string=w2132, offset (0)=5, length (rest)=10 ("length (rest)")) -> (substring=w2125:string)
          n1703 = Fract/Exp String To Number(string=w2125) -> (number=w2126:dbl)  [unwired: 3 in, 1 out]
          n1704 = Match Pattern(string=w2130, regular expression="-") -> (before substring=w2128:string)  [unwired: 1 in, 3 out]
          n1705 = case shown="10" w2127 {
            tunnel: w2126 -> [_ _ _ _ _ _ _ _ _ _ w2140 _ _ _ _ _ _ _ _ _ _ _ _ _]
            tunnel: w2128 -> [_ _ _ _ w2136 w2137 w2138 _ _ _ _ _ _ _ _ _ _ _ _ _ w2141 w2142 w2143 _]
            frame 0 {
            }
            frame 1 {
            }
            frame 2 {
            }
            frame 3 {
            }
            frame 4 {
              n1706 = local write "Com Port 1"(w2136) -> ()
            }
            frame 5 {
              n1707 = local write "Com Port 2"(w2137) -> ()
              n1708 = local write "visa due"(w2137) -> ()
            }
            frame 6 {
              n1709 = String To Path(string=w2138) -> (path=w2139:path)
              n1710 = local write "File Path"(w2139) -> ()
              "String" <- w2138
            }
            frame 7 {
            }
            frame 8 {
            }
            frame 9 {
            }
            frame 10 {
              n1711 = local write "Language Selection"(w2140) -> ()
            }
            frame 11 {
            }
            frame 12 {
            }
            frame 13 {
            }
            frame 14 {
            }
            frame 15 {
            }
            frame 16 {
            }
            frame 17 {
            }
            frame 18 {
            }
            frame 21 {
            }
            frame 22 {
              n1712 = local write "Com Port 3"(w2141) -> ()
            }
            frame 20 {
              n1713 = local write "Camera Port :"(w2142) -> ()
            }
            frame 19 {
              n1714 = local write "C3 :"(w2143) -> ()
            }
            frame 23, Default {
            }
          }
        }
      }
    }
    n1715 = Select(t=u32 2500 ("milliseconds to wait"), s=w2110, f=u32 500 ("milliseconds to wait")) -> (s? t:f=w2108:u32)
    n1716 = Multiply(x=w2113, y=w2108) -> (x*y=w2115:dbl)
    n1717 = call "Elapsed Time2"("Time Target (s)"=w2115, "Auto Reset"=TRUE) -> ("Time has Elapsed"=w2105:bool)  [unwired: 10 in, 7 out]
    n1718 = case shown="True" w2105 {
      frame False {
      }
      frame True {
        n1719 = stacked-sequence {
          frame #0 {
            # "DATA PROCESSING"
            # "115 mV/N"
            n1720 = local read "Sample Temperature"() -> (w2146:dbl)
            n1721 = local read "RH Numeric:"() -> (→"Humidity ( %RH )" →"Hum" →"Hum 2":dbl)
            n1722 = local read "FRICVALZ"() -> (w2163:dbl)
            n1723 = local read "Friction"() -> (w2149:dbl)
            n1724 = call <vilib>:"Mean PtByPt.vi"("x"=w2146, "sample length"=100) -> ("mean"=w2145:dbl)  [unwired: 2 in, 1 out]
            "TEMP 2" <- w2145
            "TEMP 3" <- w2145
            n1725 = Subtract(x=w2149, y=w2163) -> (x-y=w2158:dbl)
            "FF 2" <- w2158
            "FF 4" <- w2158
            n1726 = local read "Ambient Temperature"() -> (→"AIR TEMP":dbl)
            n1727 = local read "TEMP"() -> (w2162:dbl)
            n1728 = local write "FF 3"(w2158) -> ()
            n1729 = Compound Arithmetic op=OR("FRICVALZ 4", "FRICVALZ 3", "FRICVALZ 2") -> (w2154:bool)
            n1730 = case shown="True" w2154 {
              tunnel: w2149 -> [_ w2169]
              frame False {
              }
              frame True {
                w2168 = FALSE ("FRICVALZ")
                n1731 = local write "FRICVALZ 3"(w2168) -> ()
                n1732 = local write "FRICVALZ 2"(w2168) -> ()
                n1733 = local write "FRICVALZ 4"(w2168) -> ()
                "FRICVALZ" <- w2169
              }
            }
            n1734 = Not A Number/Path/Refnum?(number/path/refnum=w2162) -> (NaN/Path/Refnum?=w2161:bool)
            n1735 = Not A Number/Path/Refnum?(number/path/refnum=w2158) -> (NaN/Path/Refnum?=w2160:bool)
            n1736 = Divide(x=w2158, y=1.96) -> (x/y=w2155:dbl)
            n1737 = Compound Arithmetic op=OR(w2161, w2160) -> (w2159:bool)
            n1738 = Not A Number/Path/Refnum?(number/path/refnum=w2155) -> (NaN/Path/Refnum?=w2156:bool)
            n1739 = case shown="True" w2159 {
              frame False {
              }
              frame True {
                n1740 = local write "TEMP"(0.0 ("TEMP")) -> ()
                n1741 = local write "FF 2"(0.0 ("FF 2")) -> ()
                n1742 = local write "reinit"(TRUE ("reinit")) -> ()
              }
            }
            n1743 = local write "TEMP"(w2145) -> ()
            n1744 = Select(t=0.0, s=w2156, f=w2155) -> (s? t:f=w2148:dbl)
            "COF 2" <- w2148
            n1745 = local write "COF 3"(w2148) -> ()
          }
        }
      }
    }
    n1746 = Wait (ms)(milliseconds to wait=u32 50) -> ()  [unwired: 1 out]
    n1747 = local read "Quit"() -> (w2099:bool)
    "Rate" <- 2500.0 ("No of Samples")
  }
  n1748 = while {
    tunnel: [w2189] -> _
    tunnel: [w2172] -> w56
    tunnel: w1 -> [_]
    i -> [w2189]
    stop <- w2172 stop-if-true
    # "C:\\LAB-IQ-NXT\\Scar View.exe"
    n1749 = local read "OK Button 16"() -> (w2179:bool)
    n1750 = local read "Main Tab"() -> (w2173:T2)
    n1751 = local read "service 3"() -> (w2174:bool)
    n1752 = local read "OPEN 6"() -> (w2176:bool)
    n1753 = local read "EDIT 2"() -> (w2178:bool)
    n1754 = flat-sequence {
      frame #0 {
        n1755 = stacked-sequence {
          frame #0 {
            n1756 = local read "EDIT"() -> (w2667:bool)
            n1757 = case shown="False" w2667 {
              tunnel: [u8 2 ("Disabled") u8 0 ("Disabled")] -> _
              frame False {
                w2669 = FALSE
                n1758 = local write "Password"("") -> ()
                n1759 = local write "x = y?"(w2669) -> ()
                n1760 = property on="Password" class="Str"("Visible"=w2669) -> ()  [unwired: 2 in, 2 out]
              }
              frame True {
                n1761 = property on="Password" class="Str"("Visible"=TRUE) -> ()  [unwired: 2 in, 2 out]
              }
            }
            "dipl pwd" <- "@143$\n" ("dipl pwd")
          }
          frame #1 {
          }
          frame #2 {
          }
          frame #3 {
          }
          frame #4 {
            n1762 = String To Byte Array(string="Password") -> (unsigned byte array=w2680:u8[])
            n1763 = Search 1D Array(1D array=w2680, element=u8 10) -> (index of element=w2678:i32)  [unwired: 1 in]
            n1764 = Index Array(array=w2680, index=w2678) -> (element=w2679:u8)
            n1765 = Equal?(x=w2679, y=10) -> (x = y?=w2675:bool)
            n1766 = case shown="True" w2675 {
              frame False {
              }
              frame True {
                # "password"
                # "password"
                n1767 = local read "Password"() -> (w2692:string)
                n1768 = String To Byte Array(string=w2692) -> (unsigned byte array=w2695:u8[])
                n1769 = String To Byte Array(string="@143$\n") -> (unsigned byte array=w2682:u8[])
                n1770 = Array Size(array=w2695) -> (size(s)=w2691:i32)
                n1771 = Array Size(array=w2682) -> (size(s)=w2687:i32)
                n1772 = for {
                  N: w2691 -> [_]
                  tunnel: w2695 -> [w2708]
                  tunnel: [w2706] -> w2696 mode=indexing
                  tunnel: w2691 -> [w2703]
                  i -> [w2704]
                  n1773 = Decrement(x=w2703) -> (x-1=w2702:i32)
                  n1774 = Index Array(array=w2708, index=w2704) -> (element=w2707:u8)
                  n1775 = Equal?(x=w2704, y=w2702) -> (x = y?=w2701:bool)
                  n1776 = Number To Decimal String(number=w2707) -> (decimal integer string=w2705:string)  [unwired: 1 in]
                  n1777 = Select(t="", s=w2701, f="\r") -> (s? t:f=w2698:string)
                  n1778 = Concatenate Strings(w2705, w2698) -> (w2706:string)
                }
                n1779 = for {
                  N: w2687 -> [_]
                  tunnel: w2682 -> [w2719]
                  tunnel: [w2717] -> w2685 mode=indexing
                  tunnel: w2687 -> [w2714]
                  i -> [w2715]
                  n1780 = Decrement(x=w2714) -> (x-1=w2713:i32)
                  n1781 = Index Array(array=w2719, index=w2715) -> (element=w2718:u8)
                  n1782 = Equal?(x=w2715, y=w2713) -> (x = y?=w2712:bool)
                  n1783 = Number To Decimal String(number=w2718) -> (decimal integer string=w2716:string)  [unwired: 1 in]
                  n1784 = Select(t="", s=w2712, f="\r") -> (s? t:f=w2709:string)
                  n1785 = Concatenate Strings(w2716, w2709) -> (w2717:string)
                }
                n1786 = local read "file path"() -> (w2681:path)
                n1787 = call <vilib>:"Read Characters From File.vi"("file path (dialog if empty)"=w2681) -> ("character string"=w2694:string)  [unwired: 5 in, 3 out]
                "string" <- w2694
                n1788 = flat-sequence {
                  tunnel: [w2697] -> _
                  frame #0 {
                    w2697 = ""
                    n1789 = local write "Password"(w2697) -> ()
                  }
                }
                n1790 = Concatenate Strings(w2685) -> (w2686:string)
                n1791 = Concatenate Strings(w2694) -> (w2693:string)
                n1792 = Concatenate Strings(w2696) -> (w2689:string)
                n1793 = Equal?(x=w2689, y=w2693) -> (x = y?=w2684:bool)
                n1794 = Equal?(x=w2689, y=w2686) -> (x = y?=w2690:bool)
                n1795 = Or(x=w2684, y=w2690) -> (x .or. y?=→"x = y?":bool)
              }
            }
          }
        }
        n1796 = local read "x = y?"() -> (w2665:bool)
        n1797 = And(x="EDIT", y=w2665) -> (x .and. y?=w2663:bool)
        n1798 = case shown="True" w2663 {
          tunnel: [u8 2 ("Disabled") u8 0 ("Disabled")] -> w2662
          tunnel: [w2869 TRUE ("Visible")] -> w2661
          frame False {
            w2869 = FALSE ("Visible")
            n1799 = local write "EDIT 2"(w2869) -> ()
          }
          frame True {
          }
        }
        n1800 = case shown="True" "SAVE" {
          frame False {
          }
          frame True {
            n1801 = stacked-sequence {
              seq-local: [w2724 _ _] -> [_ w2865 _]
              frame #0 {
                w2720 = 0.0 ("number")
                w2721 = 0.0 ("number")
                (unwired) i16 5 ("precision (6)")
                # "[CH1]    - FF\n[CH2]   - TEMPERATURE\n[CH3]    - Humidity\n[CH4]    - AIR TEMP\n[CH5]\\- Visa Uno\n[CH6] \\- Visa Due\n[CH7]  \\- file path\n[CH8]   - Displacement Gain\n[CHA]   - Stroke Gain\n[CHB]   - Stroke PID Gain\n[CHC]   -Language Selection\n[CHD]   -Power +\n[CHE]   -Power_\n[CHF]   -Heater\n[CHG]   -Humidity Wet\n[CHH]   -Humidity Dry\n[CHI]   -Integral Time"
                n1802 = local read "Language Selection"() -> (w2767:enum16{"English", "Russian"})
                n1803 = Path To String(path="File Path") -> (string=w2783:string)
                n1804 = Number To Fractional String(number=w2720, width (-)=i16 10 ("precision (6)"), precision (6)=i16 5) -> (F-format string=w2774:string)  [unwired: 1 in]
                n1805 = Number To Fractional String(number=w2767, width (-)=i16 10 ("precision (6)"), precision (6)=i16 5) -> (F-format string=w2763:string)  [unwired: 1 in]
                n1806 = Number To Fractional String(number=w2721, width (-)=i16 10 ("precision (6)"), precision (6)=i16 5) -> (F-format string=w2757:string)  [unwired: 1 in]
                n1807 = Number To Fractional String(number=w2721, width (-)=i16 10 ("precision (6)"), precision (6)=i16 5) -> (F-format string=w2754:string)  [unwired: 1 in]
                n1808 = Number To Fractional String(number=w2721, width (-)=i16 10 ("precision (6)"), precision (6)=i16 5) -> (F-format string=w2749:string)  [unwired: 1 in]
                n1809 = Number To Fractional String(number=w2721, width (-)=i16 10 ("precision (6)"), precision (6)=i16 5) -> (F-format string=w2746:string)  [unwired: 1 in]
                n1810 = Number To Fractional String(number=w2721, width (-)=i16 10 ("precision (6)"), precision (6)=i16 5) -> (F-format string=w2741:string)  [unwired: 1 in]
                n1811 = local read "Com Port 1"() -> (w2723:refnum<visa-resource-name>)
                n1812 = local read "Com Port 2"() -> (w2722:refnum<visa-resource-name>)
                n1813 = Concatenate Strings(w2783, "\\" ("string")) -> (w2782:string)
                n1814 = Number To Fractional String(number=w2720, width (-)=i16 10 ("precision (6)"), precision (6)=i16 5) -> (F-format string=w2815:string)  [unwired: 1 in]
                n1815 = Number To Fractional String(number=w2720, width (-)=i16 10 ("precision (6)"), precision (6)=i16 5) -> (F-format string=w2814:string)  [unwired: 1 in]
                n1816 = Number To Fractional String(number=w2720, width (-)=i16 10 ("precision (6)"), precision (6)=i16 5) -> (F-format string=w2808:string)  [unwired: 1 in]
                n1817 = Number To Fractional String(number=w2720, width (-)=i16 10 ("precision (6)"), precision (6)=i16 5) -> (F-format string=w2802:string)  [unwired: 1 in]
                n1818 = Number To Fractional String(number=w2720, width (-)=i16 10 ("precision (6)"), precision (6)=i16 5) -> (F-format string=w2775:string)  [unwired: 1 in]
                n1819 = Concatenate Strings("[CHA]" ("string"), w2774, "- Stroke Gain" ("string"), "\r") -> (w2768:string)
                n1820 = Concatenate Strings("[CHC]" ("string"), w2763, "-Language Selection" ("string"), "\r") -> (w2760:string)
                n1821 = Concatenate Strings("[CHD]" ("string"), w2757, "-Power +" ("string"), "\r") -> (w2739:string)
                n1822 = Concatenate Strings("[CHG]" ("string"), w2746, "-Humidity Wet" ("string"), "\r") -> (w2736:string)
                n1823 = Concatenate Strings("[CHH]" ("string"), w2741, "-Humidity Dry" ("string"), "\r") -> (w2735:string)
                n1824 = Concatenate Strings("[CH1]" ("string"), w2815, " - FF" ("string"), "\r") -> (w2813:string)
                n1825 = Concatenate Strings("[CH2]" ("string"), w2814, " - TEMPERATURE" ("string"), "\r") -> (w2812:string)
                n1826 = Concatenate Strings("[CH3]" ("string"), w2808, " - Humidity" ("string"), "\r") -> (w2805:string)
                n1827 = Concatenate Strings("[CH4]" ("string"), w2802, " - AIR TEMP" ("string"), "\r") -> (w2798:string)
                n1828 = Concatenate Strings("[CH5]" ("string"), w2723, "- Visa Uno" ("string"), "\r") -> (w2791:string)
                n1829 = Concatenate Strings("[CH6]" ("string"), w2722, "- Visa Due" ("string"), "\r") -> (w2786:string)
                n1830 = Concatenate Strings("[CH7]" ("string"), w2782, "- file path" ("string"), "\r") -> (w2785:string)
                n1831 = Concatenate Strings("[CH8]" ("string"), w2775, "- Displacement Gain" ("string"), "\r") -> (w2778:string)
                n1832 = Concatenate Strings("[CHE]" ("string"), w2754, "-Power_" ("string"), "\r") -> (w2738:string)
                n1833 = Concatenate Strings("[CHF]" ("string"), w2749, "-Heater" ("string"), "\r") -> (w2737:string)
                n1834 = Concatenate Strings(w2813, w2812, w2805, w2798, w2791, w2786, w2785, w2778, w2768, w2760, w2739, w2738, w2737, w2736, w2735) -> (w2724:string)
                "gain" <- w2724
              }
              frame #1 {
                w2826 = 0.0 ("number")
                n1835 = local read "Camera Port :"() -> (w2829:string)
                n1836 = local read "C3 :"() -> (w2837:refnum<visa-resource-name>)
                n1837 = local read "Com Port 3"() -> (w2838:refnum<visa-resource-name>)
                n1838 = Concatenate Strings("[CH8]" ("string"), w2829, "- Visa Camera" ("string"), "\r") -> (w2828:string)
                n1839 = Concatenate Strings("[CH7]" ("string"), w2837, "- Visa Humidity" ("string"), "\r") -> (w2833:string)
                n1840 = Number To Fractional String(number=w2826, width (-)=i16 10 ("precision (6)"), precision (6)=i16 5) -> (F-format string=w2853:string)  [unwired: 1 in]
                n1841 = Concatenate Strings("[CHL]" ("string"), w2838, "- Visa humid" ("string"), "\r") -> (w2841:string)
                n1842 = Number To Fractional String(number=w2826, width (-)=i16 10 ("precision (6)"), precision (6)=i16 5) -> (F-format string=w2860:string)  [unwired: 1 in]
                n1843 = Concatenate Strings("[CHK]" ("string"), w2853, "-TEMP INTERCEPT" ("string"), "\r") -> (w2849:string)
                n1844 = Concatenate Strings("[SNO]" ("string"), "" ("string"), "-" ("string"), "\r") -> (w2846:string)
                n1845 = Concatenate Strings("[CHJ]" ("string"), w2860, "-AIR TEMP INTERCEPT" ("string"), "\r") -> (w2850:string)
                n1846 = String To Path(string="C:\\LAB-IQ\\calibrate WO 2465.dcf") -> (path=w2839:path)
                n1847 = Concatenate Strings(w2865, w2850, w2849, w2846, w2841, w2833, w2828) -> (w2864:string)
                n1848 = call <vilib>:"Write Characters To File.vi"("append to file? (new file:F)"=FALSE, "character string"=w2864, "file path (dialog if empty)"=w2839) -> ()  [unwired: 2 in, 1 out]
              }
              frame #2 {
                n1849 = local write "Lan flag"(0.0 ("Lan flag")) -> ()
                n1850 = local write "conststatus"(0.0 ("rpm value : 2")) -> ()
                n1851 = local write "SAVE"(FALSE ("OK Button 14")) -> ()
              }
            }
          }
        }
        n1852 = property on="EDIT 2" class="Bool (strict)"("Visible"=w2661) -> ()  [unwired: 2 in, 2 out]
        n1853 = property on="SAVE" class="Bool (strict)"("Visible"=w2661) -> ()  [unwired: 2 in, 2 out]
        n1854 = property on="visa due" class="CmbBox"("Disabled"=w2662) -> ()  [unwired: 2 in, 2 out]
        n1855 = property on="File Path" class="Path"("Disabled"=w2662) -> ()  [unwired: 2 in, 2 out]
        n1856 = property on="Language Selection" class="Enum (strict)"("Visible"=w2661) -> ()  [unwired: 2 in, 2 out]
        n1857 = property on="SPEED OUT:" class="DigNum (strict)"("Disabled"=w2662) -> ()  [unwired: 2 in, 2 out]
      }
    }
    n1858 = local read "RUN"() -> (w2188:bool)
    n1859 = local read "RUN"() -> (w2186:bool)
    n1860 = case shown="True" "EDIT 3" {
      frame False {
      }
      frame True {
        n1861 = local write "EDIT 3"(FALSE ("EDIT 3")) -> ()
        n1862 = local write "Main Tab"(T2."About" ("Main Tab")) -> ()
      }
    }
    n1863 = case shown="False" w2188 {
      frame False {
        n1864 = local read "stopT"() -> (w2876:bool)
        n1865 = case shown="True" w2876 {
          frame False {
          }
          frame True {
            n1866 = local write "stopT"(FALSE) -> ()
          }
        }
      }
      frame True {
        "stopT" <- TRUE
      }
    }
    n1867 = case shown="False" w2186 {
      frame False {
      }
      frame True {
      }
    }
    n1868 = case shown="True" w2178 {
      frame False {
        n1869 = property on="Password 2" class="Str"("Visible"=FALSE) -> ()  [unwired: 2 in, 2 out]
        n1870 = local write "Password 2"("" ("Password")) -> ()
      }
      frame True {
        n1871 = property on="Password 2" class="Str"("Visible"=TRUE) -> ()  [unwired: 2 in, 2 out]
        n1872 = Equal?(x="Password 2", y="HFRR1234") -> (x = y?=w2201:bool)
        n1873 = case shown="True" w2201 {
          tunnel: "Password 2" -> [w2204 _]
          frame False {
            n1874 = String Length(string=w2204) -> (length=w2205:i32)
            n1875 = Greater Than 0?(x=w2205) -> (x > 0?=w2203:bool)
            n1876 = case shown="False" w2203 {
              frame False {
                n1877 = property on="Password 2" class="Str"("Caption.Text"="Password (Advance Setting)") -> ()  [unwired: 2 in, 2 out]
              }
              frame True {
                n1878 = property on="Password 2" class="Str"("Caption.Text"="Incorrect Password!") -> ()  [unwired: 2 in, 2 out]
              }
            }
          }
          frame True {
            n1879 = local write "EDIT 2"(FALSE ("EDIT 2")) -> ()
            n1880 = local write "Password 2"("" ("Password")) -> ()
            n1881 = local write "Main Tab"(T2."Advance" ("Main Tab")) -> ()
            n1882 = local write "Main Dashboard Buttons"(T1."Advance" ("Main Dashboard Buttons")) -> ()
          }
        }
      }
    }
    n1883 = case shown="True" "Prog Uno" {
      frame False {
      }
      frame True {
        n1884 = stacked-sequence {
          frame #0 {
            n1885 = Delete(path (use dialog)=path "C:/LAB-IQ-NXT/UNOCOMPILE.bat" ("working directory")) -> ()  [unwired: 4 in, 3 out]
          }
          frame #1 {
            n1886 = local read "Com Port 1"() -> (w2643:refnum<visa-resource-name>)
            n1887 = Concatenate Strings("cmd.exe /c \"mode " ("command line"), w2643, ":1200,n,8,1\"\n" ("command line")) -> (w2648:string)
            n1888 = Concatenate Strings(w2648, "CD\\\nCD WinDucom\navrdude -C avrdude.conf -v -patmega328p -carduino -P" ("command line"), w2643, " -b115200 -D -Uflash:w:UNO_V20.hex:i\n" ("command line"), "\r") -> (w2650:string)
            "STR" <- w2650
            n1889 = call <vilib>:"Write Characters To File.vi"("append to file? (new file:F)"=FALSE, "character string"=w2650, "file path (dialog if empty)"=path "C:/LAB-IQ/UNOCOMPILE.bat" ("working directory")) -> ()  [unwired: 2 in, 1 out]
          }
